vi "ClimbWeight.vi"   [LabVIEW 2013]
uses:
  Sally_Framework_2014/State_Machine_Enum.ctl
  <vilib>/Rock Robotics/WPI/Solenoid/WPI_SolenoidValue.ctl
  Robot Global Data.vi
  <vilib>/Rock Robotics/WPI/Solenoid/WPI_SolenoidSetEnum.vi
types:
  T1 = typedef "State_Machine_Enum.ctl" = enum16{"Idle", "Start", "Do", "Stop", "Init"}
  T2 = typedef "WPI_SolenoidValue.ctl" = enum16{"Off", "On", "Forward", "Reverse"}
  T3 = typedef "WPI_SolenoidDevRef.ctl" = cluster{"DevStatus":errorcluster, "Solenoid Module":T4, "Forward Solenoid Channel":T5, "Reverse Solenoid Channel":T5}
  T4 = typedef "FPGA_TypedefSolenoidModule.ctl" = enum16{"Solenoid Module 1", "Solenoid Module 2"}
  T5 = typedef "WPI_SolenoidChannel.ctl" = enum8{"Solenoid 1", "Solenoid 2", "Solenoid 3", "Solenoid 4", "Solenoid 5", "Solenoid 6", "Solenoid 7", "Solenoid 8", "Invalid"}
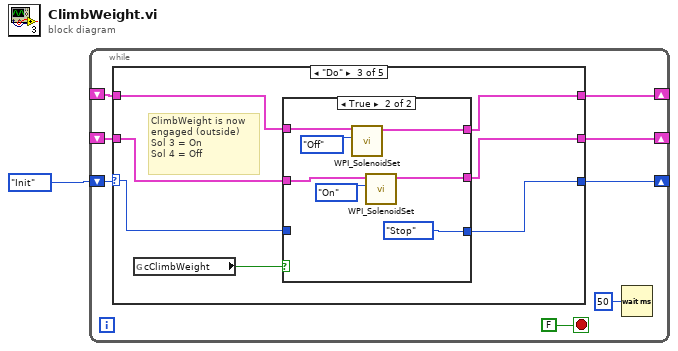
[diagram p0: block diagram]
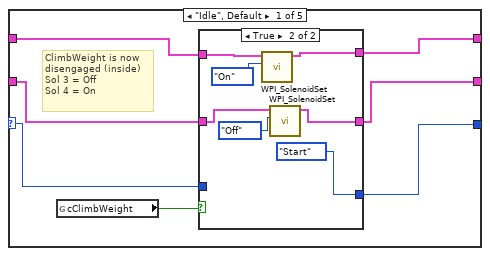
[diagram p2: hidden frame]
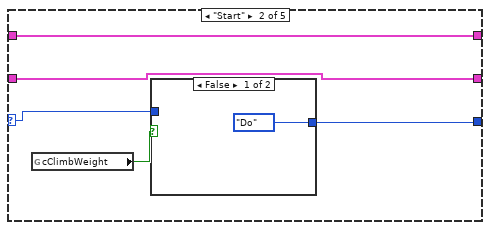
[diagram p4: hidden frame]
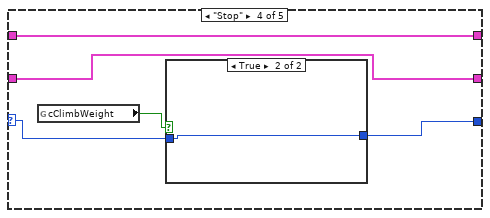
[diagram p7: hidden frame]
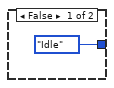
[diagram p8: hidden frame]
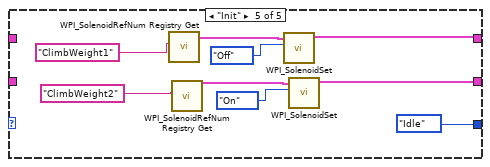
[diagram p9: hidden frame]
diagram:
  n1 = while {
    shift-right: [w8] -> _
    shift-left: State_Machine_Enum."Init" ("State") -> [w9]
    shift-right: [w7] -> _
    shift-left: _ -> [w6]
    shift-right: [w3] -> _
    shift-left: _ -> [w2]
    stop <- FALSE stop-if-true
    n2 = case shown="\"Do\"" w9 {
      selector: w9 -> [w13 w29 w37 w54 _]
      tunnel: [w14 w30 w38 w55 State_Machine_Enum."Idle" ("State")] -> w8
      tunnel: [w15 w31 w39 w53 w64] -> w7
      tunnel: w6 -> [w16 w31 w40 w53 _]
      tunnel: [w11 w28 w35 w52 w60] -> w3
      tunnel: w2 -> [w12 w28 w36 w52 _]
      frame "Idle", Default {
        # "ClimbWeight is now\ndisengaged (inside)\nSol 3 = Off\nSol 4 = On"
        n3 = global read "Robot Global Data.vi" "cClimbWeight"() -> (w10:bool)
        n4 = case shown="True" w10 {
          tunnel: w16 -> [w18 w26]
          tunnel: [w18 w25] -> w15
          tunnel: [w19 State_Machine_Enum."Start" ("State")] -> w14
          tunnel: w13 -> [w19 _]
          tunnel: w12 -> [w17 w21]
          tunnel: [w17 w20] -> w11
          frame False {
          }
          frame True {
            n5 = call-poly <vilib>:"WPI_SolenoidSet.vi"("Value"=WPI_SolenoidValue."On", "SolenoidDevRef"=w26) -> ("SolenoidDevRef"=w25:T3)  [unwired: 8 in, 1 out]
            n6 = call-poly <vilib>:"WPI_SolenoidSet.vi"("Value"=WPI_SolenoidValue."Off", "SolenoidDevRef"=w21) -> ("SolenoidDevRef"=w20:T3)  [unwired: 8 in, 1 out]
          }
        }
      }
      frame "Start" {
        n7 = global read "Robot Global Data.vi" "cClimbWeight"() -> (w27:bool)
        n8 = case shown="False" w27 {
          tunnel: [State_Machine_Enum."Do" ("State") w33] -> w30
          tunnel: w29 -> [_ w33]
          frame False {
          }
          frame True {
          }
        }
      }
      frame "Do" {
        # "ClimbWeight is now\nengaged (outside)\nSol 3 = On\nSol 4 = Off"
        n9 = global read "Robot Global Data.vi" "cClimbWeight"() -> (w34:bool)
        n10 = case shown="True" w34 {
          tunnel: w40 -> [w43 w50]
          tunnel: [w43 w49] -> w39
          tunnel: [w42 State_Machine_Enum."Stop" ("State")] -> w38
          tunnel: w37 -> [w42 _]
          tunnel: w36 -> [w41 w45]
          tunnel: [w41 w44] -> w35
          frame False {
          }
          frame True {
            n11 = call-poly <vilib>:"WPI_SolenoidSet.vi"("Value"=WPI_SolenoidValue."Off", "SolenoidDevRef"=w50) -> ("SolenoidDevRef"=w49:T3)  [unwired: 8 in, 1 out]
            n12 = call-poly <vilib>:"WPI_SolenoidSet.vi"("Value"=WPI_SolenoidValue."On", "SolenoidDevRef"=w45) -> ("SolenoidDevRef"=w44:T3)  [unwired: 8 in, 1 out]
          }
        }
      }
      frame "Stop" {
        n13 = global read "Robot Global Data.vi" "cClimbWeight"() -> (w51:bool)
        n14 = case shown="True" w51 {
          tunnel: [State_Machine_Enum."Idle" ("State") w57] -> w55
          tunnel: w54 -> [_ w57]
          frame False {
          }
          frame True {
          }
        }
      }
      frame "Init" {
        n15 = call <vilib>:"WPI_SolenoidRefNum Registry Get.vi"("refnum name"="ClimbWeight1") -> ("SolenoidDevRef"=w65:T3)  [unwired: 9 in, 1 out]
        n16 = call <vilib>:"WPI_SolenoidRefNum Registry Get.vi"("refnum name"="ClimbWeight2") -> ("SolenoidDevRef"=w61:T3)  [unwired: 9 in, 1 out]
        n17 = call-poly <vilib>:"WPI_SolenoidSet.vi"("Value"=WPI_SolenoidValue."Off", "SolenoidDevRef"=w65) -> ("SolenoidDevRef"=w64:T3)  [unwired: 8 in, 1 out]
        n18 = call-poly <vilib>:"WPI_SolenoidSet.vi"("Value"=WPI_SolenoidValue."On", "SolenoidDevRef"=w61) -> ("SolenoidDevRef"=w60:T3)  [unwired: 8 in, 1 out]
      }
    }
    n19 = Wait (ms)(milliseconds to wait=u32 50) -> ()  [unwired: 1 out]
  }
